vi "Set HW Interface Digital Outputs.vi"(8 "error in (no error)":errorcluster, 10 "Digital Outputs":T1, 11 "Grips Robot in":refnum<class "Grips Robot.lvclass">) -> (0 "error out":errorcluster, 3 "Grips Robot out":refnum<class "Grips Robot.lvclass">)   [LabVIEW 2013, in "Grips Robot.lvclass"]
uses:
  Grips Robot.lvclass
  Hardware Interface/BoolArrayWithName.ctl
  Grips Robot.lvclass/Grips Robot.ctl
  Hardware Interface/Hardware Interface.lvclass/Hardware Interface.ctl
  Hardware Interface/Hardware Interface.lvclass
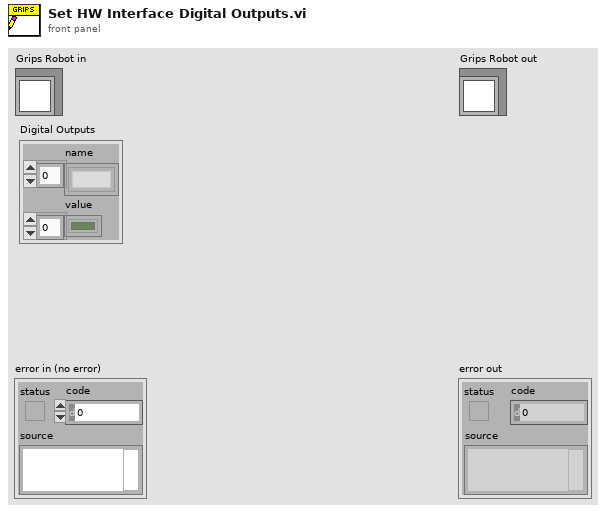
[diagram p1: front panel]
types:
  T1 = typedef "Hardware Interface.lvclass/BoolArrayWithName.ctl" = cluster{"name":string[], "value":bool[]}
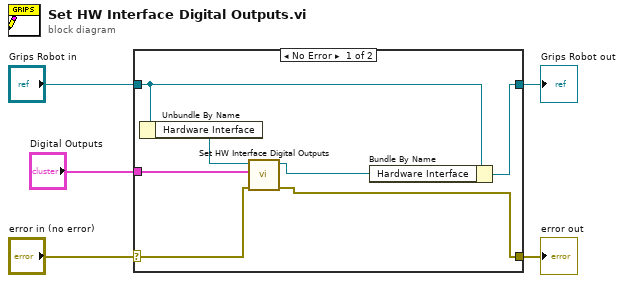
[diagram p0: block diagram]
diagram:
  n1 = case shown="No Error" "error in (no error)" {
    selector: "error in (no error)" -> [w9 w13]
    tunnel: [w10 w13] -> w4
    tunnel: [w12 w14] -> w2
    tunnel: "Grips Robot in" -> [w8 w14]
    tunnel: "Digital Outputs" -> [w6 _]
    frame No Error {
      n2 = Unbundle By Name(w8) -> ("Hardware Interface"=w7:refnum<class "Hardware Interface.lvclass">)
      n3 = call "Set HW Interface Digital Outputs.vi"("error in (no error)"=w9, "Digital Outputs"=w6, "Hardware Interface in"=w7) -> ("error out"=w10:errorcluster, "Hardware Interface out"=w11:refnum<class "Hardware Interface.lvclass">)  [unwired: 7 in]
      n4 = Bundle By Name(cluster=w8, "Hardware Interface"=w11) -> (w12:refnum<class "Grips Robot.lvclass">)
    }
    frame Error {
    }
  }
  "error out" <- w4
  "Grips Robot out" <- w2
